vi "2ndOrderTF.vi"(7 "Initialize?":bool, 9 "Denominator (a1, a2)":T1=[0.0, 0.0], 10 "Numerator (b0, b1, b2)":T2=[0.0, 0.0, 0.0], 11 "Ctrl Effort In":fxp<+/-,25,5>) -> (3 "Ctrl Effort Out":fxp<+/-,25,5>)   [LabVIEW 2020, in "Controller.lvlib"]
doc: "<b>2nd-order Discrete Transfer Function implementation </b>\n\nImplements, u(k) = b0*e(k) + b1*e(k-1) + b2*e(k-2) - a1*u(k-1) - a2*u(k-2)\n\nSet parameters, Num = b0, b1, b2 and Den = a1, a2\n\nTF implemented: (b0 z^2 + b1 z + b2 ) / (z^2 + a1 z + a2)"
uses:
  Controller.lvlib
  TypeDefs/2ndOrderTFnum.ctl
  TypeDefs/2ndOrderTFden.ctl
  <vilib>/Platform/TimedLoop/XDataNode/timing_clust.ctl
  <vilib>/Platform/TimedLoop/XDataNode/nitl_modes.ctl
  <vilib>/Platform/TimedLoop/XDataNode/wakeup.ctl
  <vilib>/rvi/Emulation/niFpgaSctlEmulationGetInTimedLoop.vi
  <vilib>/rvi/Emulation/niFpgaEmulationReportErrorSimple.vi
  <vilib>/rvi/Emulation/niFpgaGetClockAttributes.vi
  <vilib>/rvi/Emulation/niFpgaCriticalErrorInLSC.vi
  <vilib>/Platform/TimedLoop/XDataNode/XDataNode.xnode
  <vilib>/rvi/FXPMathLib/FxpMul/XNode/nifxpmath_Multiplier.xnode
  <vilib>/rvi/FXPMathLib/FxpAdd/XNode/nifxpmath_Add.xnode
  <vilib>/rvi/FXPMathLib/FxpSub/XNode/nifxpmath_Sub.xnode
  <vilib>/Platform/TimedLoop/XDataNode/XDNodeRunTimeDep.lvlib
  <vilib>/rvi/FXPMathLib/sim/FxpSim.dll
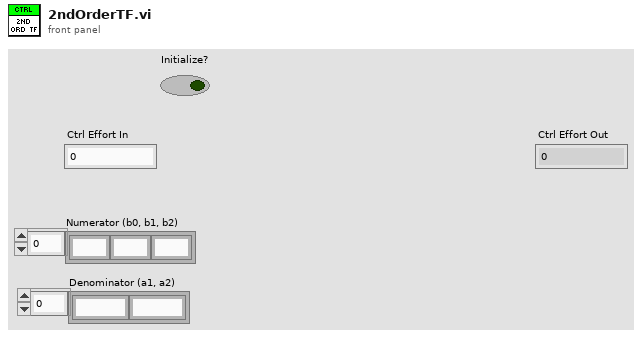
[diagram p1: front panel]
types:
  T1 = typedef "Controller.lvlib/2ndOrderTFden.ctl" = fxp<+/-,28,2>[]
  T2 = typedef "Controller.lvlib/2ndOrderTFnum.ctl" = fxp<+/-,28,2>[]
  T3 = typedef "XDNodeRunTimeDep.lvlib/timing_clust.ctl" = cluster{"Expected End [f-1]":u64, "Actual End [f-1]":u64, "Finished Late? [f-1]":bool, "Expected End [i-1]":u64, "Actual End [i-1]":u64, "Finished Late? [i-1]":bool, "Expected Start [i]":u64, "Actual Start [i]":u64, "Expected Start [f]":u64, "Actual Start [f]":u64, "Source Name":string, "Structure Name":string, "Period":i64, "Deadline":i64, "Offset":i64, "Start":i64, "Priority":i32, "Timeout":i32, "Mode":T4, "Wakeup Reason":T5, "Error":errorcluster, "Source Type":string, "Secondary Source Type":string, "Global End Time":u64, "Global Start Time":u64, "Frame Duration":u64, "Iteration Duration":u64, "Assigned CPU":i32, "I/O Scan Engine Mode":u32}
  T4 = typedef "XDNodeRunTimeDep.lvlib/nitl_modes.ctl" = enum32{"No Change", "Process missed periods, maintain original phase", "Discard missed periods, maintain original phase", "Process missed periods, ignore original phase", "Discard missed periods, ignore original phase"}
  T5 = typedef "XDNodeRunTimeDep.lvlib/wakeup.ctl" = enum32{"Normal", "Aborted", "Asynchronous wakeup", "Timing source error", "Timed loop error", "Timeout"}
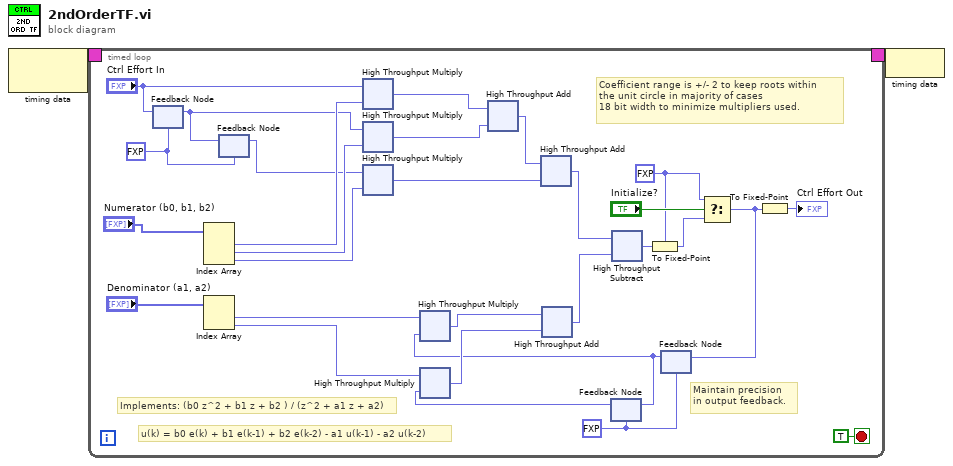
[diagram p0: block diagram]
diagram:
  n1 = node-c288() -> (w2:T3)  [unwired: 1 in]
  n2 = timed-loop {
    timing: w2 -> [_]
    timing-out: [_] -> w1
    stop <- TRUE stop-if-true
    w27 = fxp<+/-,25,5> 0.0 ("t")
    w29 = fxp<+/-,42,5> 0.0 ("t")
    w9 = fxp<+/-,42,5> 0.0 ("t")
    # "Implements: (b0 z^2 + b1 z + b2 ) / (z^2 + a1 z + a2)"
    # "Coefficient range is +/- 2 to keep roots within \nthe unit circle in majority of cases\n18 bit width to minimize multipliers used."
    # "Maintain precision \nin output feedback."
    # "u(k) = b0 e(k) + b1 e(k-1) + b2 e(k-2) - a1 u(k-1) - a2 u(k-2)"
    n3 = feedback-in #1("Ctrl Effort In") -> ()
    n4 = feedback #1(w27) -> (w24:fxp<+/-,25,5>)
    n5 = Index Array(array="Numerator (b0, b1, b2)") -> (element #1=w26:fxp<+/-,28,2>, element #2=w25:fxp<+/-,28,2>, element #3=w23:fxp<+/-,28,2>)  [unwired: 3 in]
    n6 = Index Array(array="Denominator (a1, a2)") -> (element #1=w21:fxp<+/-,28,2>, element #2=w19:fxp<+/-,28,2>)  [unwired: 2 in]
    n7 = feedback #2(w27) -> (w22:fxp<+/-,25,5>)
    n8 = feedback-in #2(w24) -> ()
    n9 = xnode ("High Throughput Multiply")("x"="Ctrl Effort In", "y"=w26) -> ("x*y"=w18:fxp<+/-,53,7>)
    n10 = xnode ("High Throughput Multiply")("x"=w24, "y"=w25) -> ("x*y"=w17:fxp<+/-,53,7>)
    n11 = xnode ("High Throughput Multiply")("x"=w22, "y"=w23) -> ("x*y"=w16:fxp<+/-,53,7>)
    n12 = xnode ("High Throughput Add")("x"=w18, "y"=w17) -> ("x+y"=w15:fxp<+/-,54,8>)
    n13 = xnode ("High Throughput Add")("x"=w15, "y"=w16) -> ("x+y"=w12:fxp<+/-,55,9>)
    n14 = feedback #3(w29) -> (w20:fxp<+/-,42,5>)
    n15 = xnode ("High Throughput Multiply")("x"=w19, "y"=w20) -> ("x*y"=w13:fxp<+/-,44,7>)
    n16 = feedback #4(w29) -> (w3:fxp<+/-,42,5>)
    n17 = xnode ("High Throughput Multiply")("x"=w21, "y"=w3) -> ("x*y"=w14:fxp<+/-,44,7>)
    n18 = xnode ("High Throughput Add")("x"=w14, "y"=w13) -> ("x+y"=w11:fxp<+/-,45,8>)
    n19 = feedback-in #3(w3) -> ()
    n20 = xnode ("High Throughput Subtract")("x"=w12, "y"=w11) -> ("x-y"=w10:fxp<+/-,56,10>)
    n21 = To Fixed-Point(fixed-point type=w9, number=w10) -> (fixed-point=w8:fxp<+/-,42,5>)
    n22 = Select(t=w9, s="Initialize?", f=w8) -> (s? t:f=w4:fxp<+/-,42,5>)
    n23 = feedback-in #4(w4) -> ()
    n24 = To Fixed-Point(number=w4) -> (fixed-point=→"Ctrl Effort Out":fxp<+/-,25,5>)  [unwired: 1 in]
  }
  n25 = node-c288(w1) -> ()
